vi "Get Next Step.vi"(8 "error in (no error)":errorcluster, 11 "Actor in":refnum<class "Actor.lvclass">) -> (0 "error out":errorcluster, 1 "Parameter":variant, 2 "Step":string, 3 "Actor out":refnum<class "Actor.lvclass">, 4 "Reply Channel":refnum<notifier>)   [LabVIEW 2015, in "Actor.lvclass"]
uses:
  Actor.lvclass
  Messaging/Message/Message.lvclass
  Actor.lvclass/Actor.ctl
  <userlib>/_OpenG.lib/string/string.llb/Trim Whitespace (String)__ogtk.vi
  Sequencer/Sequencer.lvclass
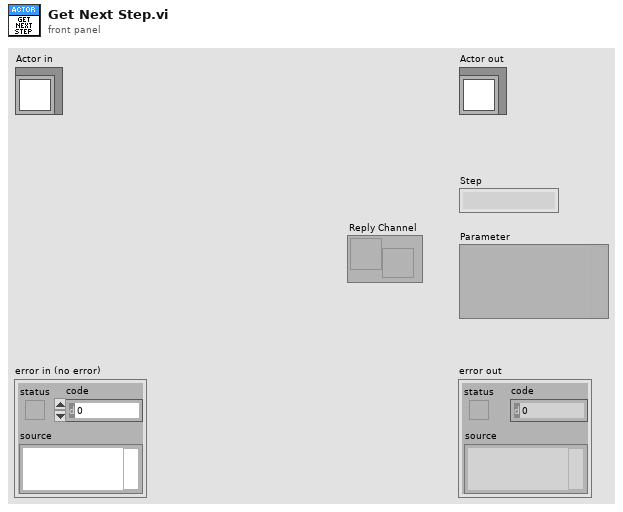
[diagram p1: front panel]
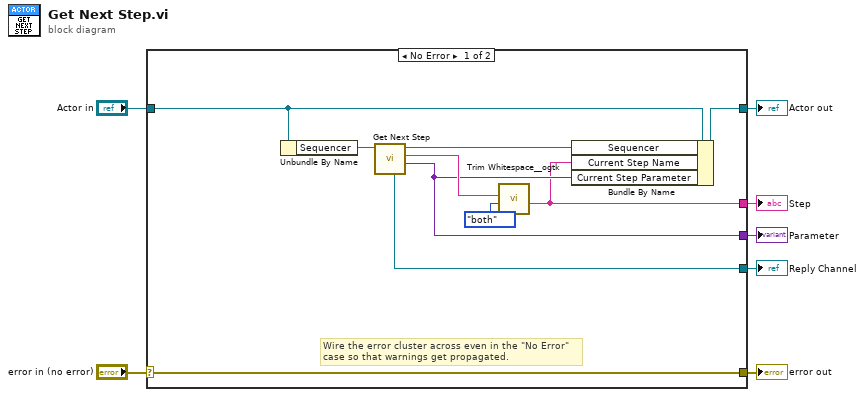
[diagram p0: block diagram]
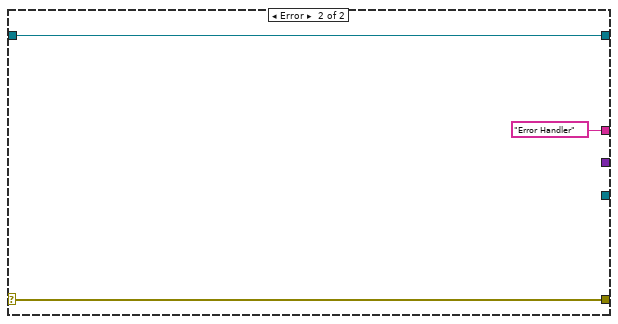
[diagram p2: hidden frame]
diagram:
  n1 = case shown="No Error" "error in (no error)" {
    selector: "error in (no error)" -> [w17 w20]
    tunnel: [w17 w20] -> w6
    tunnel: [w13 w19] -> w4
    tunnel: "Actor in" -> [w14 w19]
    tunnel: [w9 "Error Handler" ("Step")] -> w3
    tunnel: [w10 _] -> w2
    tunnel: [w8 _] -> w1
    frame No Error {
      # "Wire the error cluster across even in the \"No Error\"\ncase so that warnings get propagated."
      n2 = Unbundle By Name(w14) -> ("Sequencer"=w16:refnum<class "Sequencer.lvclass">)
      n3 = call "Get Next Step.vi"("Sequencer in"=w16) -> ("Parameter"=w10:variant, "Step"=w11:string, "Sequencer out"=w12:refnum<class "Sequencer.lvclass">, "Reply Channel"=w8:refnum<notifier>)  [unwired: 6 in, 1 out]
      n4 = call-poly <userlib>:"Trim Whitespace__ogtk.vi"("Remove (leading and trailing)"=enum16{"leading", "trailing", "both"}."both", "String in"=w11) -> ("String out"=w9:string)  [unwired: 5 in]
      n5 = Bundle By Name(cluster=w14, "Sequencer"=w12, "Current Step Name"=w9, "Current Step Parameter"=w10) -> (w13:refnum<class "Actor.lvclass">)
    }
    frame Error {
    }
  }
  "error out" <- w6
  "Actor out" <- w4
  "Step" <- w3
  "Parameter" <- w2
  "Reply Channel" <- w1
